vi "Jinv_quart.vi"(1 "eta":dbl[](array[numeric])) -> (0 "Jinv":T1)   [LabVIEW 2014]
uses:
  <vilib>/Analysis/Matrix/Datatypes/RealMatrix.ctl
  <vilib>/Analysis/_algsub.llb/Real PseudoInverse Matrix.vi
  TransformationMatrixQuaternions.vi
  RotationMatrixQuaternions.vi
  <vilib>/imath/engines/lvmath2/RunTimeEngine/RowToken/NIMS_RowToken_M_M.vi
  <instcachedir>/0/NIMS_RowToken_M_M_4C96C156B57B4BCFA08E125188784392.lvgen/NIMS_RowToken_M_M_4C96C156B57B4BCFA08E125188784392_004.vi
  <vilib>/imath/engines/lvmath2/RunTimeEngine/MatrixToken/NIMS_MatrixToken_M_M.vi
  <instcachedir>/0/NIMS_MatrixToken_M_M_F8DD6808CBBD42C5992E1D2201A8964A.lvgen/NIMS_MatrixToken_M_M_F8DD6808CBBD42C5992E1D2201A8964A_004.vi
  <vilib>/imath/engines/lvmath2/RunTimeEngine/ErrorHandling/NIMS_Create Error From Enums.vi
  <vilib>/imath/engines/lvmath2/RunTimeEngine/NodeEndStatement/NIMS_NodeEndStatement_Output.vi
  <instcachedir>/0/NIMS_NodeEndStatement_Output_53EC0D466D134D7ABD903AC30B43404B.lvgen/NIMS_NodeEndStatement_Output_53EC0D466D134D7ABD903AC30B43404B_002.vi
  <vilib>/imath/engines/lvmath2/RunTimeEngine/ErrorHandling/NIMS_Finalize Error.vi
  <vilib>/Analysis/Matrix/Numeric/Conversions/Array To Matrix - RA2.vi
  <vilib>/Analysis/Matrix/NI_Matrix.lvlib
  <vilib>/Analysis/NI_AALPro.lvlib
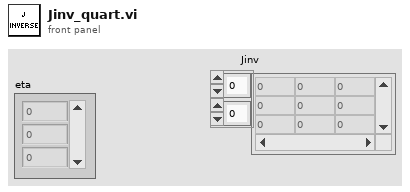
[diagram p1: front panel]
types:
  T1 = typedef "NI_Matrix.lvlib/RealMatrix.ctl" = dbl[][]
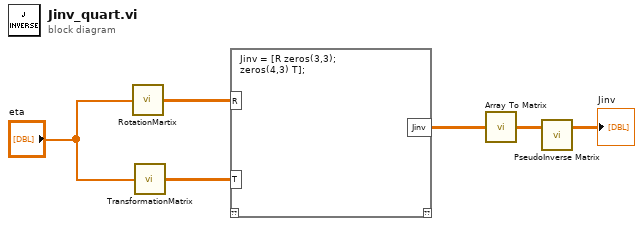
[diagram p0: block diagram]
diagram:
  n1 = call-poly "RotationMartix.vi"("Eta_q"="eta") -> ("R"=w4:dbl[][])
  n2 = call-poly "TransformationMatrix.vi"("Eta_q"="eta") -> ("T_q"=w5:dbl[][])
  n3 = mathscript code="Jinv = [R zeros(3,3);\nzeros(4,3) T];"("R"=w4, "T"=w5) -> ("Jinv"=w3:dbl[][])  [unwired: 1 in, 1 out]
  n4 = call-poly <vilib>:"Array To Matrix.vi"("Real 2D Array"=w3) -> ("Real Matrix"=w2:T1)
  n5 = call-poly <vilib>:"PseudoInverse Matrix.vi"("Input Matrix"=w2) -> ("PseudoInverse Matrix"=→"Jinv":T1)  [unwired: 1 in, 1 out]
